vi "Data trimming.vi"(8 "error in":errorcluster, 9 "#A-lines to save":i32=300, 10 "#B-lines":i32=2048, 11 "2D Array in":sgl[][](array[numeric])) -> (0 "error out":errorcluster, 2 "time":dbl, 3 "output array":sgl[](array[numeric]))   [LabVIEW 2018]
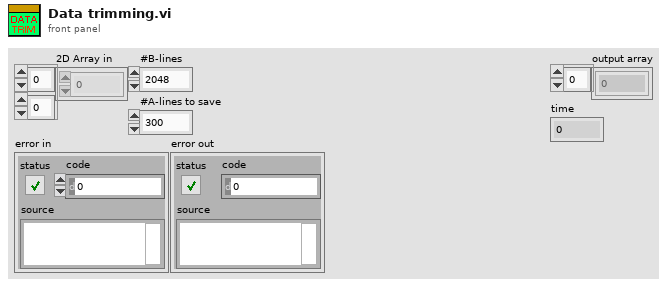
[diagram p1: front panel]
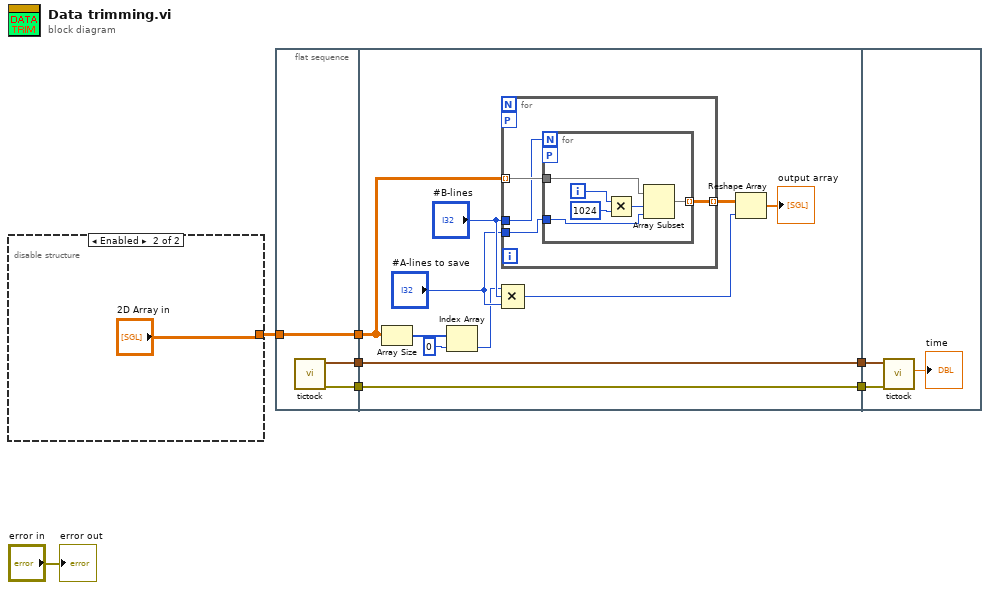
[diagram p0: block diagram]
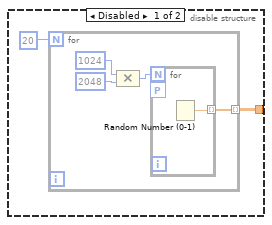
[diagram p2: hidden frame]
diagram:
  n1 = disable-structure shown="Enabled" {
    disable-tunnel: [w8 "2D Array in"] -> w6
    frame Disabled {
      n2 = for {
        N: 20 -> [_]
        tunnel: [w10] -> w8 mode=indexing
        n3 = Compound Arithmetic op=MULTIPLY(1024, 2048) -> (w11:i32)
        n4 = for {
          N: w11 -> [_]
          tunnel: [w14] -> w10 mode=indexing
          workers-P: _ -> [_]
          n5 = Random Number (0-1)() -> (number: 0 to 1=w14:dbl)
        }
      }
    }
    frame Enabled {
    }
  }
  n6 = flat-sequence {
    tunnel: w6 -> [w18]
    tunnel: [w18] -> w5
    tunnel: [w17] -> w3
    tunnel: [w16] -> w1
    tunnel: w5 -> [w24]
    tunnel: [w23] -> w4
    tunnel: w3 -> [w23]
    tunnel: [w22] -> w2
    tunnel: w1 -> [w22]
    tunnel: w4 -> [w42]
    tunnel: w2 -> [w41]
    frame #0 {
      n7 = call "tictock.vi"() -> ("error out"=w16:errorcluster, "seconds since 1Jan1904"=w17:timestamp)  [unwired: 9 in, 1 out]
    }
    frame #1 {
      n8 = Array Size(array=w24) -> (size(s)=w27:i32[])
      n9 = Index Array(array=w27, index=0) -> (element=w25:i32)
      n10 = for {
        tunnel: w24 -> [w33] mode=indexing
        workers-P: _ -> [_]
        tunnel: [w32] -> w21 mode=indexing
        tunnel: "#B-lines" -> [w31]
        tunnel: "#A-lines to save" -> [w30]
        n11 = for {
          N: w31 -> [_]
          tunnel: w33 -> [w36]
          workers-P: _ -> [_]
          tunnel: [w35] -> w32 mode=indexing
          tunnel: w30 -> [w34]
          i -> [w39]
          n12 = Multiply(x=w39, y=1024) -> (x*y=w37:i32)
          n13 = Array Subset(array=w36, index=w37, length=w34) -> (w35:sgl[])
        }
      }
      n14 = Compound Arithmetic op=MULTIPLY(w25, "#B-lines", "#A-lines to save") -> (w20:i32)
      n15 = Reshape Array(w21, w20) -> (→"output array":sgl[])
    }
    frame #2 {
      n16 = call "tictock.vi"("error in (no error)"=w41, "seconds since 1Jan1904 2"=w42) -> ("Numeric"=→"time":dbl)  [unwired: 7 in, 2 out]
    }
  }
  "error out" <- "error in"
